vi "Write Serial Configuration.vi"(8 "error in (no error)":errorcluster, 10 "Serial Configuration":T1={"Baud Rate"=9600, "Parity"=0, "Data Bits"=8, "Stop Bits"=10, "Flow Control"=0} {"Flow Control" items=["None", "XON/XOFF", "RTS/CTS", "XON/XOFF & RTS/CTS", "DTR/DSR", "XON/XOFF & DTR/DSR"]; "Stop Bits" items=["1.0"=10, "1.5"=15, "2.0"=20]; "Data Bits" items=["7"=7, "8"=8]; "Parity" items=["None", "Odd", "Even", "Mark", "Space"]; "Baud Rate" items=["300"=300, "600"=600, "1200"=1200, "2400"=2400, "4800"=4800, "9600"=9600, "19200"=19200]}, 11 "Motor-GWInstek in":refnum<class "Motor-GWInstek.lvclass">) -> (0 "error out":errorcluster, 3 "Motor-GWInstek out":refnum<class "Motor-GWInstek.lvclass">)   [LabVIEW 2013, in "PowderDeposition.lvlib" / "Motor-GWInstek.lvclass"]
uses:
  Motor-GWInstek.lvclass
  Motor-GWInstek.lvclass/Motor-GWInstek.ctl
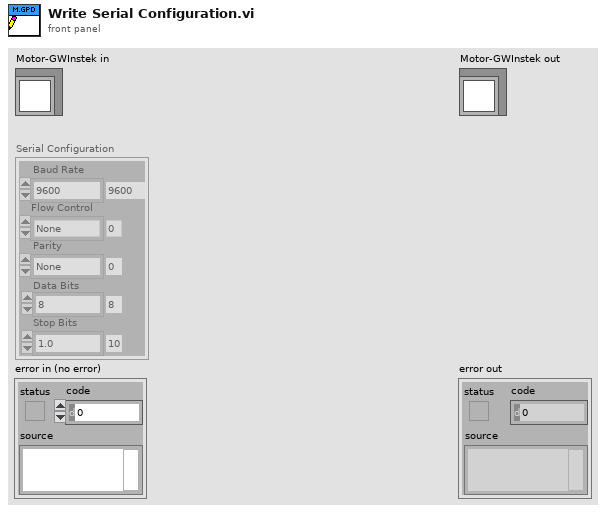
[diagram p1: front panel]
types:
  T1 = cluster{"Baud Rate":u32, "Parity":u16, "Data Bits":u16, "Stop Bits":u16, "Flow Control":u16}
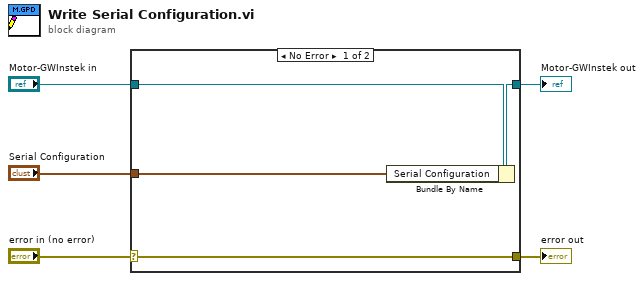
[diagram p0: block diagram]
diagram:
  n1 = case shown="No Error" "error in (no error)" {
    selector: "error in (no error)" -> [w9 w10]
    tunnel: [w9 w10] -> w4
    tunnel: [w7 w11] -> w2
    tunnel: "Motor-GWInstek in" -> [w8 w11]
    tunnel: "Serial Configuration" -> [w6 _]
    frame No Error {
      n2 = Bundle By Name(cluster=w8, "Serial Configuration"=w6) -> (w7:refnum<class "Motor-GWInstek.lvclass">)
    }
    frame Error {
    }
  }
  "error out" <- w4
  "Motor-GWInstek out" <- w2
